vi "ingresaMediciones.vi"(8 "error in (no error)":errorcluster, 9 "Selection Start":T1, 11 "Prueba05 in":refnum<class "Prueba05.lvclass">) -> (0 "error out":errorcluster, 3 "Prueba05 out":refnum<class "Prueba05.lvclass">)   [LabVIEW 2019, in "Prueba05.lvclass"]
uses:
  Prueba05.lvclass
  <vilib>/Utility/miscctls.llb/LVRowAndColumnTypeDef.ctl
  Prueba05.lvclass/Prueba05.ctl
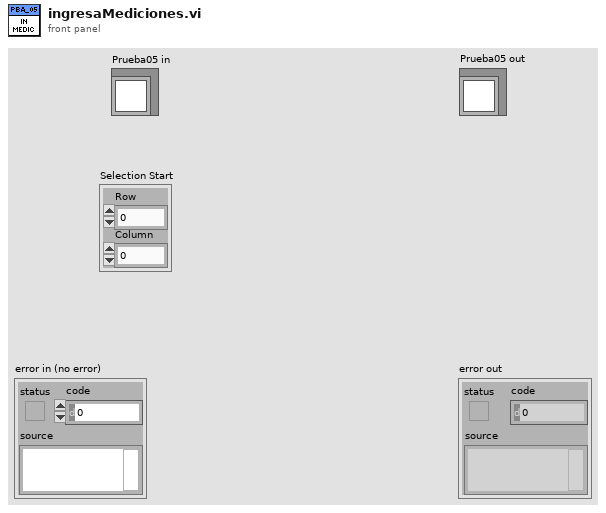
[diagram p1: front panel]
types:
  T1 = typedef "LVRowAndColumnTypeDef.ctl" = cluster{"Row":i32, "Column":i32}
  T2 = cluster{"Medido":dbl, "error":dbl, "Ref":dbl, "Incert_exp":dbl, "Tol+":dbl, "Tol-":dbl, "fila":i32}
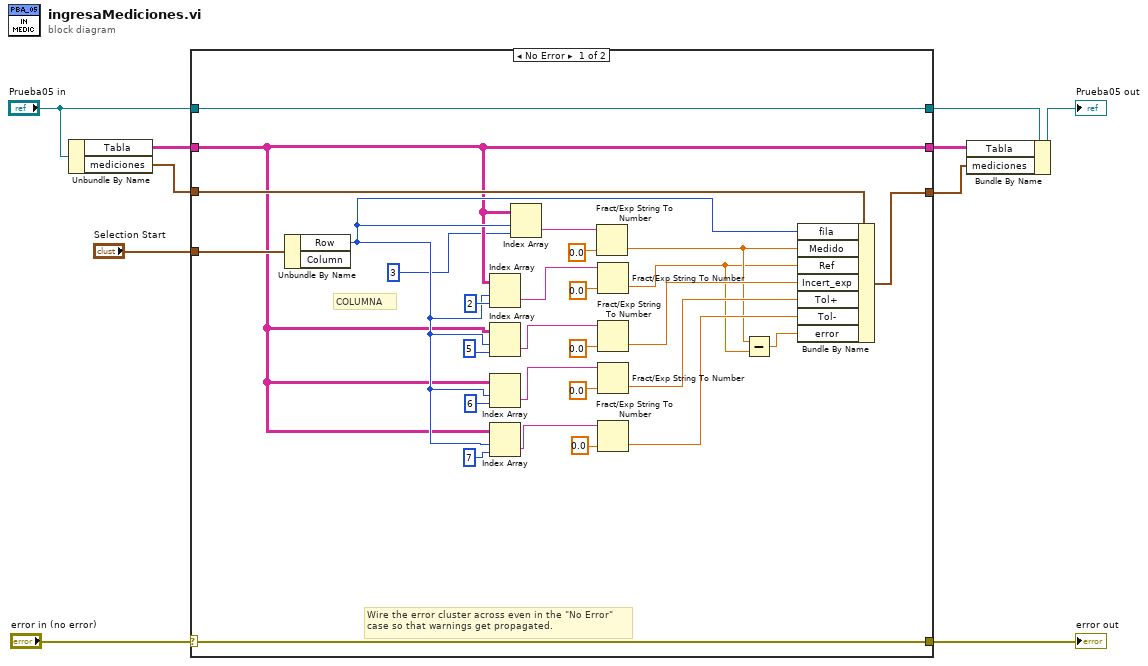
[diagram p0: block diagram]
diagram:
  n1 = Unbundle By Name("Prueba05 in") -> ("Tabla"=w6:string[][], "mediciones"=w5:T2)
  n2 = case shown="No Error" "error in (no error)" {
    selector: "error in (no error)" -> [w37 w42]
    tunnel: [w37 w42] -> w9
    tunnel: [w38 w41] -> w8
    tunnel: "Prueba05 in" -> [w38 w41]
    tunnel: w6 -> [w13 w40]
    tunnel: w5 -> [w19 w39]
    tunnel: [w13 w40] -> w3
    tunnel: [w18 w39] -> w2
    tunnel: "Selection Start" -> [w14 _]
    frame No Error {
      # "COLUMNA"
      # "Wire the error cluster across even in the \"No Error\"\ncase so that warnings get propagated."
      n3 = Unbundle By Name(w14) -> ("Row"=w20:i32)  [unwired: 1 out]
      n4 = Index Array(array=w13, index (row)=w20, index (col)=2 ("disabled index (col)")) -> (element=w34:string)
      n5 = Index Array(array=w13, index (row)=w20, index (col)=5 ("index (row)")) -> (element=w30:string)
      n6 = Index Array(array=w13, index (row)=w20, index (col)=6 ("disabled index (col)")) -> (element=w21:string)
      n7 = Index Array(array=w13, index (row)=w20, index (col)=7 ("index (row)")) -> (element=w24:string)
      n8 = Index Array(array=w13, index (row)=w20, index (col)=3 ("Column")) -> (element=w12:string)
      n9 = Fract/Exp String To Number(string=w12, default (0 dbl)=0.0) -> (number=w17:dbl)  [unwired: 2 in, 1 out]
      n10 = Fract/Exp String To Number(string=w34, default (0 dbl)=0.0) -> (number=w16:dbl)  [unwired: 2 in, 1 out]
      n11 = Fract/Exp String To Number(string=w30, default (0 dbl)=0.0) -> (number=w29:dbl)  [unwired: 2 in, 1 out]
      n12 = Fract/Exp String To Number(string=w21, default (0 dbl)=0.0) -> (number=w22:dbl)  [unwired: 2 in, 1 out]
      n13 = Fract/Exp String To Number(string=w24, default (0 dbl)=0.0) -> (number=w23:dbl)  [unwired: 2 in, 1 out]
      n14 = Subtract(x=w17, y=w16) -> (x-y=w15:dbl)
      n15 = Bundle By Name(cluster=w19, "fila"=w20, "Medido"=w17, "Ref"=w16, "Incert_exp"=w29, "Tol+"=w22, "Tol-"=w23, "error"=w15) -> (w18:T2)
    }
    frame Error {
    }
  }
  "error out" <- w9
  n16 = Bundle By Name(cluster=w8, "Tabla"=w3, "mediciones"=w2) -> (→"Prueba05 out":refnum<class "Prueba05.lvclass">)
